vi "out.vi"(11 "Outputs":T1) -> ()   [LabVIEW 2012]
uses:
  util/Outputs.ctl
  climber/climber_outputs.ctl
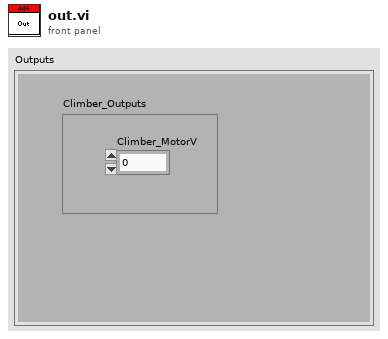
[diagram p1: front panel]
types:
  T1 = typedef "Outputs.ctl" = cluster{"Climber_Outputs":T2}
  T2 = typedef "climber_outputs.ctl" = cluster{"Climber_MotorV":dbl}
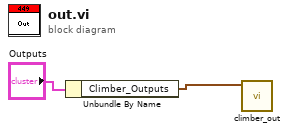
[diagram p0: block diagram]
diagram:
  n1 = Unbundle By Name("Outputs") -> ("Climber_Outputs"=w1:T2)
  n2 = call "climber_out.vi"("Climber_Outputs"=w1) -> ()  [unwired: 11 in]
